vi "Load Report.vi"(8 "error in (no error)":errorcluster, 11 "HIJ Vision File Viewer in":refnum<class "HIJ Vision File Viewer.lvclass">) -> (0 "error out":errorcluster, 3 "HIJ Vision File Viewer out":refnum<class "HIJ Vision File Viewer.lvclass">)   [LabVIEW 2014, in "HIJ Vision File Viewer.lvlib" / "HIJ Vision File Viewer.lvclass"]
uses:
  HIJ Vision File Viewer.lvclass
  HIJ Vision Display/HIJ Vision Display/HIJ Vision Display.lvclass/HIJ Vision Display.ctl
  HIJ Vision File Viewer.lvclass/HIJ Vision File Viewer.ctl
  Analyze Actor/Analyze Actor Messages/Load Parameters Msg/Load Parameters Msg.lvclass/Load Parameters Msg.ctl
  <vilib>/ActorFramework/Message Enqueuer/Message Enqueuer.lvclass/Message Enqueuer.ctl
  HIJ Vision Display/HIJ Vision Display/Read Image Source Name.vi
  HIJ Vision Display/HIJ Vision Display/Read WorkDir.vi
  HIJ Vision Display/HIJ Vision Display/Read Analyze Actor.vi
  <vilib>/ActorFramework/Message Enqueuer/Enqueue.vi
  <vilib>/ActorFramework/Message Priority Queue/Priority Enqueue.vi
  <vilib>/ActorFramework/Message Enqueuer/Message Enqueuer.lvclass
  Analyze Actor/Analyze Actor Messages/Load Parameters Msg/Load Parameters Msg.lvclass
  HIJ Vision Display/HIJ Vision Display/HIJ Vision Display.lvclass
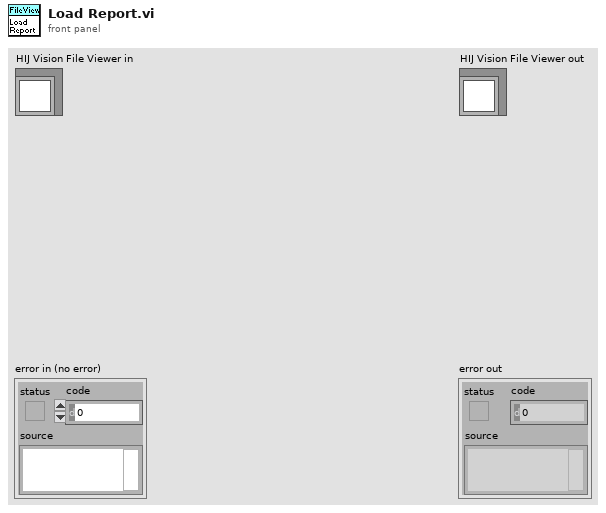
[diagram p1: front panel]
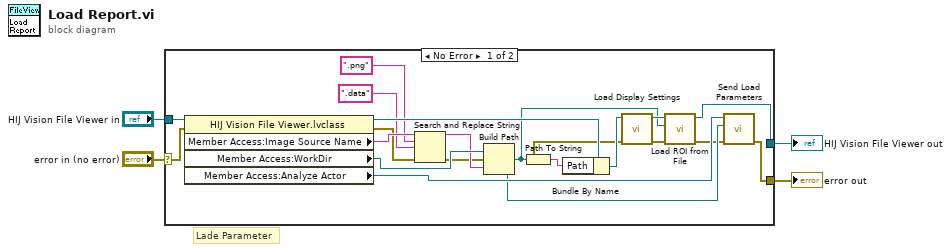
[diagram p0: block diagram]
diagram:
  # "Lade Parameter"
  n1 = case shown="No Error" "error in (no error)" {
    selector: "error in (no error)" -> [w6 w25]
    tunnel: [w15 w25] -> w3
    tunnel: [w11 w24] -> w1
    tunnel: "HIJ Vision File Viewer in" -> [w23 w24]
    frame No Error {
      n2 = property class="HIJ Vision File Viewer.lvclass"(reference=w23, error in=w6) -> (reference out=w22:refnum<class "HIJ Vision File Viewer.lvclass">, error out=w7:errorcluster, "Member Access:Image Source Name"=w21:string, "Member Access:WorkDir"=w18:path, "Member Access:Analyze Actor"=w16:refnum<class "Message Enqueuer.lvclass">)
      n3 = Search and Replace String(input string=w21, search string=".png", replace string=".data" ("search string"), error in=w7) -> (result string=w17:string, error out=w5:errorcluster)  [unwired: 4 in, 2 out]
      n4 = Build Path(base path=w18, name or relative path=w17) -> (appended path=w10:path)
      n5 = Path To String(path=w10) -> (string=w14:string)
      n6 = Bundle By Name(cluster=w22, "Path"=w14) -> (w12:refnum<class "HIJ Vision File Viewer.lvclass">)
      n7 = call-dynamic "Load Display Settings.vi"("error in (no error)"=w5, "AF IMAQ Display in"=w12) -> ("error out"=w9:errorcluster, "AF IMAQ Display out"=w13:refnum<class "HIJ Vision File Viewer.lvclass">)  [unwired: 8 in]
      n8 = call "Load ROI from File.vi"("error in (no error)"=w9, "Report File"=w10, "IMAQ Display in"=w13) -> ("error out"=w8:errorcluster, "IMAQ Display out"=w11:refnum<class "HIJ Vision File Viewer.lvclass">)  [unwired: 7 in]
      n9 = call "Send Load Parameters.vi"("error in (no error)"=w8, "Resource"=w10, "Message Enqueuer"=w16) -> ("error out"=w15:errorcluster)  [unwired: 7 in, 1 out]
    }
    frame Error {
    }
  }
  "error out" <- w3
  "HIJ Vision File Viewer out" <- w1
